vi "Close.vi"(8 "error in (no error)":errorcluster, 11 "HAL.TCP in":refnum<class "HAL.TCP.lvclass">) -> (0 "error out":errorcluster, 3 "HAL.TCP out":refnum<class "HAL.TCP.lvclass">)   [LabVIEW 2019, in "HAL.TCP.lvclass"]
uses:
  HAL.TCP.lvclass
  HAL.TCP.lvclass/HAL.TCP.ctl
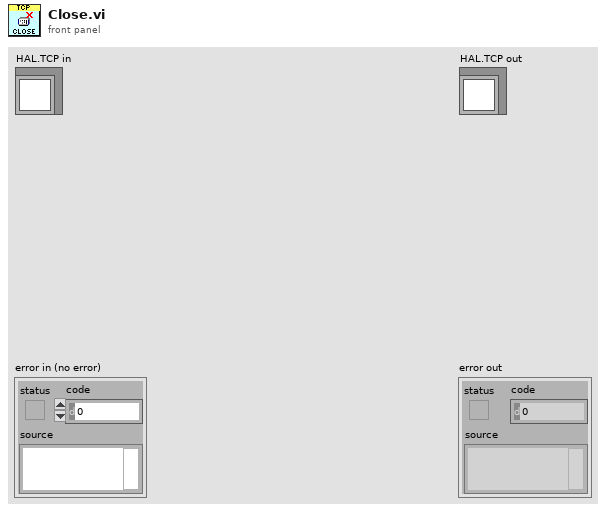
[diagram p1: front panel]
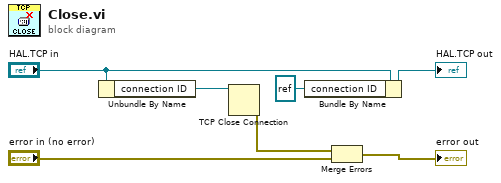
[diagram p0: block diagram]
diagram:
  n1 = Unbundle By Name("HAL.TCP in") -> ("connection ID"=w5:refnum<k5>)
  n2 = TCP Close Connection(connection ID=w5) -> (error out=w2:errorcluster)  [unwired: 2 in, 1 out]
  n3 = Bundle By Name(cluster="HAL.TCP in", "connection ID"=refnum<k5> refnum) -> (→"HAL.TCP out":refnum<class "HAL.TCP.lvclass">)
  n4 = Merge Errors(w2, "error in (no error)") -> (→"error out":errorcluster)
